vi "Write Active target.vi"(10 "Active targets":string[](array[string]), 11 "SolutionBuilder in":refnum<class "SolutionBuilder.lvclass">) -> (3 "SolutionBuilder out":refnum<class "SolutionBuilder.lvclass">)   [LabVIEW 2019, in "SolutionBuilder.lvlib" / "SolutionBuilder.lvclass"]
uses:
  SolutionBuilder.lvclass
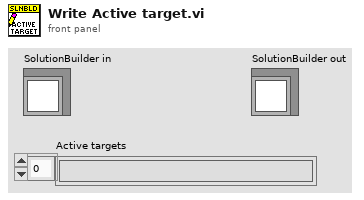
[diagram p1: front panel]
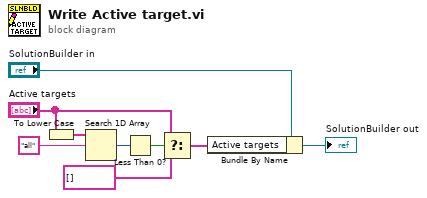
[diagram p0: block diagram]
diagram:
  n1 = To Lower Case(string="Active targets") -> (all lower case string=w6:string[])
  n2 = Search 1D Array(1D array=w6, element="all") -> (index of element=w5:i32)  [unwired: 1 in]
  n3 = Less Than 0?(x=w5) -> (x < 0?=w4:bool)
  n4 = Select(t="Active targets", s=w4, f=string[] []) -> (s? t:f=w1:string[])
  n5 = Bundle By Name(cluster="SolutionBuilder in", "Active targets"=w1) -> (→"SolutionBuilder out":refnum<class "SolutionBuilder.lvclass">)
